vi "Launch Devices.vi"(11 "gController in":refnum<class "gController.lvclass">) -> (3 "gController out":refnum<class "gController.lvclass">)   [LabVIEW 2016, in "Controller.lvlib" / "gController.lvclass"]
uses:
  gController.lvclass
  C:/Program Files (x86)/National Instruments/LabVIEW 2016/vi.lib/MSR Consulting, LLC/General Reuse/SuperActor/SuperActor.lvclass
  <vilib>/MSR Consulting, LLC/Devices/DAQ Device/Device/Device.lvclass
  C:/Program Files (x86)/National Instruments/LabVIEW 2016/vi.lib/ActorFramework/Actor/Actor.lvclass
  <vilib>/MSR Consulting, LLC/General Reuse/Session APIs/File Access/Config Data/Config Data.lvclass
  <vilib>/MSR Consulting, LLC/Devices/Alicats/Alicat Device.lvclass
  C:/Program Files (x86)/National Instruments/LabVIEW 2016/vi.lib/MSR Consulting, LLC/Devices/Configurable Device/Configurable Device.lvclass
  Messages/Update Device Configuration/Update Device Config MSG.lvclass
  C:/Program Files (x86)/National Instruments/LabVIEW 2016/vi.lib/MSR Consulting, LLC/Devices/DAQ Device/Messages/Device Configuration/Get Serialized Device Configuration MSG.lvclass
  Messages/Initialize Device SP MSG/Initialize Device SP MSG.lvclass
  C:/Program Files (x86)/National Instruments/LabVIEW 2016/vi.lib/MSR Consulting, LLC/Devices/DAQ Device/Messages/Generic CVT Init/Generic Init CVT Message.lvclass
  <vilib>/MSR Consulting, LLC/Devices/Vaisala/Vaisala.lvclass
  Messages/Update Controller Data MSG/Update gController Data MSG.lvclass
  C:/Program Files (x86)/National Instruments/LabVIEW 2016/vi.lib/MSR Consulting, LLC/General Reuse/Generic Update Data MSG/Generic Update Data MSG.lvclass
  PPT/PPT.lvclass
  <vilib>/MSR Consulting, LLC/General Reuse/SuperActor/SuperActor.lvclass/SuperActor.ctl
  <vilib>/MSR Consulting, LLC/Devices/Configurable Device/Configurable Device.lvclass/Configurable Device.ctl
  <vilib>/MSR Consulting, LLC/Devices/DAQ Device/Device/Device.lvclass/Device.ctl
  <vilib>/MSR Consulting, LLC/Devices/Configurable Device/Write ID.vi
  <vilib>/MSR Consulting, LLC/Devices/Configurable Device/Accessors/Write Config Section.vi
  <vilib>/MSR Consulting, LLC/Devices/DAQ Device/Device/Write Configurable Device.vi
  <vilib>/MSR Consulting, LLC/Devices/DAQ Device/Device/Write Update Period.vi
  <vilib>/MSR Consulting, LLC/Devices/DAQ Device/Device/Write Update Data MSG.vi
  <vilib>/MSR Consulting, LLC/Devices/DAQ Device/Device/Write Dvc Cfg MSG.vi
  <vilib>/MSR Consulting, LLC/Devices/DAQ Device/Device/Write Init CVT MSG.vi
  <vilib>/MSR Consulting, LLC/General Reuse/SuperActor/Write ID.vi
  <vilib>/MSR Consulting, LLC/General Reuse/SuperActor/Read Config Session.vi
  <vilib>/MSR Consulting, LLC/General Reuse/Session APIs/File Access/Config Data/Read Array/Read String Array.vi
  <vilib>/MSR Consulting, LLC/General Reuse/Session APIs/_Session Fwk/Session - Root.lvclass
  <vilib>/MSR Consulting, LLC/General Reuse/SuperActor/SuperActor.lvclass
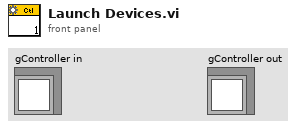
[diagram p1: front panel]
types:
  T1 = typedef "Session - Root.lvclass/Session Handle.ctl" = refnum<data-value>
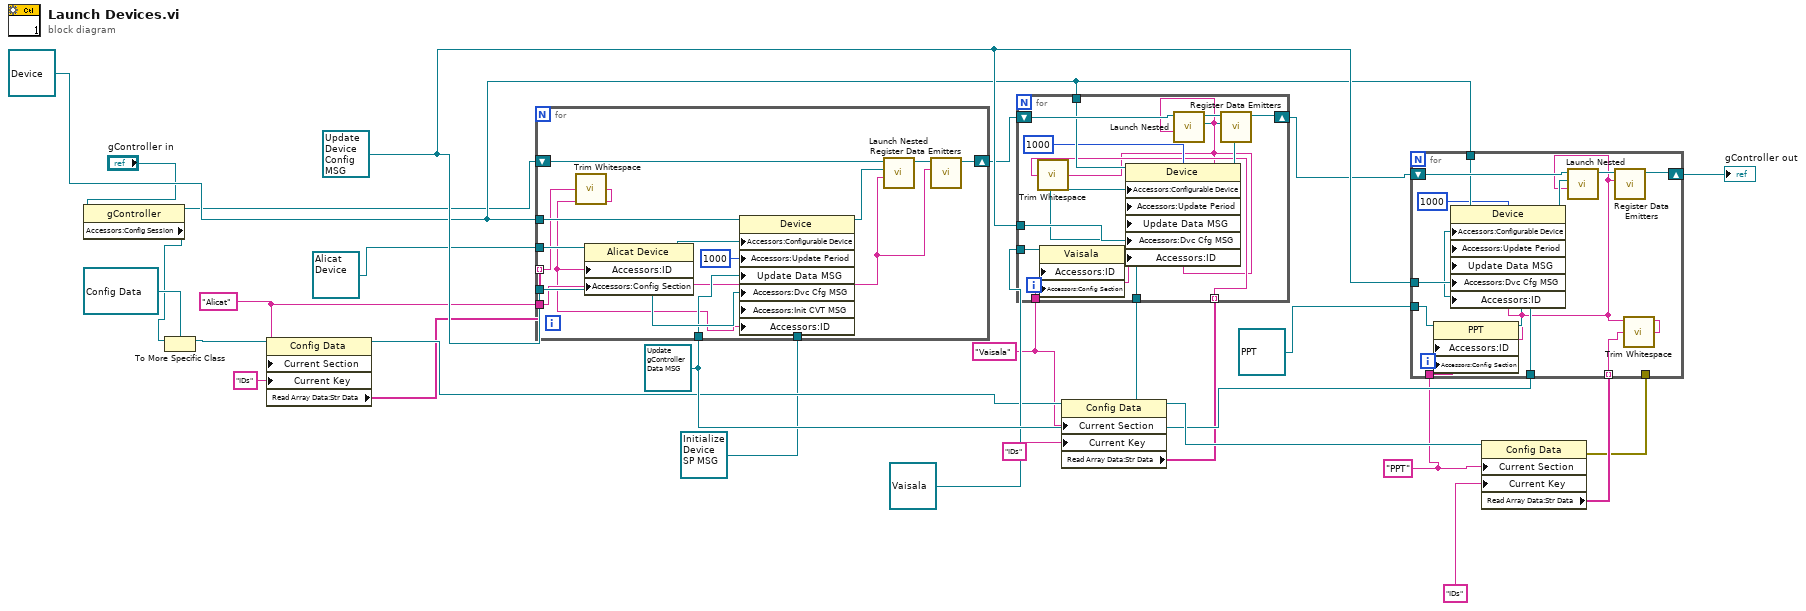
[diagram p0: block diagram]
diagram:
  w4 = "PPT" ("Current Section")
  w24 = refnum<class "Update gController Data MSG.lvclass"> refnum ("Controller.lvlib:Update gController Data MSG.lvclass")
  w3 = "Vaisala" ("Current Section")
  w23 = refnum<class "Update Device Config MSG.lvclass"> refnum ("Controller.lvlib:Update Device Config MSG.lvclass")
  w2 = "Alicat" ("Current Section")
  w7 = refnum<class "Device.lvclass"> refnum ("DAQ Device.lvlib:Device")
  n1 = property class="gController"(reference="gController in") -> (reference out=w5:refnum<class "gController.lvclass">, "Accessors:Config Session"=w9:T1)  [unwired: 1 in, 1 out]
  n2 = To More Specific Class(target class=refnum<data-value> refnum, reference=w9) -> (specific class reference=w11:refnum<data-value>)  [unwired: 1 in, 1 out]
  n3 = property class="Config Data"(reference=w11, "Current Section"=w2, "Current Key"="IDs") -> (reference out=w16:refnum<data-value>, "Read Array Data:Str Data"=w1:string[])  [unwired: 1 in, 1 out]
  n4 = for {
    tunnel: refnum<class "Alicat Device.lvclass"> refnum ("Alicat Lib.lvlib:Alicat Device") -> [w41]
    tunnel: w1 -> [w29] mode=indexing
    tunnel: w7 -> [w39]
    shift-right: [w35] -> w15
    shift-left: w5 -> [w36]
    tunnel: w23 -> [w33]
    tunnel: refnum<class "Initialize Device SP MSG.lvclass"> refnum ("Controller.lvlib:Initialize Alicat SP MSG") -> [w32]
    tunnel: w24 -> [w31]
    tunnel: w2 -> [w30]
    n5 = call <vilib>:"Trim Whitespace.vi"("string"=w29) -> ("trimmed string"=w28:string)  [unwired: 1 in]
    n6 = property class="Alicat Device"(reference=w41, "Accessors:ID"=w28, "Accessors:Config Section"=w30) -> (reference out=w40:refnum<class "Alicat Device.lvclass">)  [unwired: 1 in, 1 out]
    n7 = property class="Device"(reference=w39, "Accessors:Configurable Device"=w40, "Accessors:Update Period"=1000 ("Update Period"), "Update Data MSG"=w31, "Accessors:Dvc Cfg MSG"=w33, "Accessors:Init CVT MSG"=w32, "Accessors:ID"=w28) -> (reference out=w37:refnum<class "Device.lvclass">)  [unwired: 1 in, 1 out]
    n8 = call <vilib>:"Launch Nested.vi"("ID"=w28, "Nested Actor"=w37, "SuperActor in"=w36) -> ("SuperActor out"=w38:refnum<class "gController.lvclass">)  [unwired: 6 in, 2 out]
    n9 = call "Register Data Emitters.vi"("Emitter"=w28, "gController in"=w38) -> ("gController out"=w35:refnum<class "gController.lvclass">)  [unwired: 8 in, 1 out]
  }
  n10 = property class="Config Data"(reference=w16, "Current Section"=w3, "Current Key"="IDs") -> (reference out=w25:refnum<data-value>, "Read Array Data:Str Data"=w18:string[])  [unwired: 1 in, 1 out]
  n11 = for {
    shift-right: [w52] -> w20
    shift-left: w15 -> [w53]
    tunnel: w18 -> [w43] mode=indexing
    tunnel: w7 -> [w51]
    tunnel: w24 -> [w49]
    tunnel: w23 -> [w48]
    tunnel: refnum<class "Vaisala.lvclass"> refnum ("Vaisala Library.lvlib:Vaisala") -> [w46]
    tunnel: w3 -> [w44]
    n12 = call <vilib>:"Trim Whitespace.vi"("string"=w43) -> ("trimmed string"=w42:string)  [unwired: 1 in]
    n13 = property class="Vaisala"(reference=w46, "Accessors:ID"=w42, "Accessors:Config Section"=w44) -> (reference out=w45:refnum<class "Vaisala.lvclass">)  [unwired: 1 in, 1 out]
    n14 = property class="Device"(reference=w51, "Accessors:Configurable Device"=w45, "Accessors:Update Period"=1000 ("Update Period"), "Update Data MSG"=w49, "Accessors:Dvc Cfg MSG"=w48, "Accessors:ID"=w42) -> (reference out=w47:refnum<class "Device.lvclass">)  [unwired: 1 in, 1 out]
    n15 = call <vilib>:"Launch Nested.vi"("ID"=w42, "Nested Actor"=w47, "SuperActor in"=w53) -> ("SuperActor out"=w54:refnum<class "gController.lvclass">)  [unwired: 6 in, 2 out]
    n16 = call "Register Data Emitters.vi"("Emitter"=w42, "gController in"=w54) -> ("gController out"=w52:refnum<class "gController.lvclass">)  [unwired: 8 in, 1 out]
  }
  n17 = property class="Config Data"(reference=w25, "Current Section"=w4, "Current Key"="IDs") -> (error out=w8:errorcluster, "Read Array Data:Str Data"=w27:string[])  [unwired: 1 in, 1 out]
  n18 = for {
    shift-right: [w65] -> w21
    shift-left: w20 -> [w66]
    tunnel: w27 -> [w56] mode=indexing
    tunnel: w7 -> [w64]
    tunnel: w24 -> [w62]
    tunnel: w23 -> [w61]
    tunnel: refnum<class "PPT.lvclass"> refnum ("PPT Library.lvlib:PPT") -> [w59]
    tunnel: w8 -> [_]
    tunnel: w4 -> [w57]
    n19 = call <vilib>:"Trim Whitespace.vi"("string"=w56) -> ("trimmed string"=w55:string)  [unwired: 1 in]
    n20 = property class="PPT"(reference=w59, "Accessors:ID"=w55, "Accessors:Config Section"=w57) -> (reference out=w58:refnum<class "PPT.lvclass">)  [unwired: 1 in, 1 out]
    n21 = property class="Device"(reference=w64, "Accessors:Configurable Device"=w58, "Accessors:Update Period"=1000 ("Update Period"), "Update Data MSG"=w62, "Accessors:Dvc Cfg MSG"=w61, "Accessors:ID"=w55) -> (reference out=w60:refnum<class "Device.lvclass">)  [unwired: 1 in, 1 out]
    n22 = call <vilib>:"Launch Nested.vi"("ID"=w55, "Nested Actor"=w60, "SuperActor in"=w66) -> ("SuperActor out"=w67:refnum<class "gController.lvclass">)  [unwired: 6 in, 2 out]
    n23 = call "Register Data Emitters.vi"("Emitter"=w55, "gController in"=w67) -> ("gController out"=w65:refnum<class "gController.lvclass">)  [unwired: 8 in, 1 out]
  }
  "gController out" <- w21
